vi "Read TDM Event Data.vi"() -> ()   [LabVIEW 2023]
doc: "Reads the data written by the Write TDM Event Data.vi example."
uses:
  <vilib>/Platform/storage/lvStorage.llb/_openFunction.ctl
  <vilib>/Platform/storage/lvStorage.llb/_openStorageWithRootAutoDetect.vi
  <vilib>/Platform/storage/lvStorage.llb/xStorage/xStorageSupp/ErrorOut.vi
  <vilib>/Platform/storage/lvStorage.llb/_queryPropPoly.vi
  <vilib>/Platform/storage/lvStorage.llb/_queryPropString.vi
  <vilib>/Platform/storage/lvStorage.llb/_queryGenericObjects.vi
  <vilib>/Platform/storage/lvStorage.llb/_loadAllDdt.vi
  <vilib>/Platform/storage/lvStorage.llb/_loadAllString.vi
  <vilib>/Platform/storage/Storage.llb/Get Object Info.vi
  <vilib>/Platform/storage/Storage.llb/__closeStorageFromObject.vi
  <vilib>/Platform/storage/lvStorage.llb/xStorage/Open Data Storage/Open Data Storage.xnode
  <vilib>/Platform/storage/lvStorage.llb/xStorage/Read Data/Read Data.xnode
  <vilib>/Platform/storage/lvStorage.llb/xStorage/Close Data Storage/Close Data Storage.xnode
panel:
  out "Events":string[][](table)
  out "Data":dynamicdata(graph)
  out "Histogram Results":dynamicdata(graph)
  # "Overview: Demonstrates the use of the DataPlugin Express VIs to read event data from a TDM file.\nRequirements: Windows\nInstructions:\n1. Make sure you have already run Write TDM Event Data.vi.\n2. Run this VI. The contents of the TDM file will be displayed below.\n3. Delete the TDM file (located at [LabVIEW Data]\\Example Event File.tdm) when you are done."
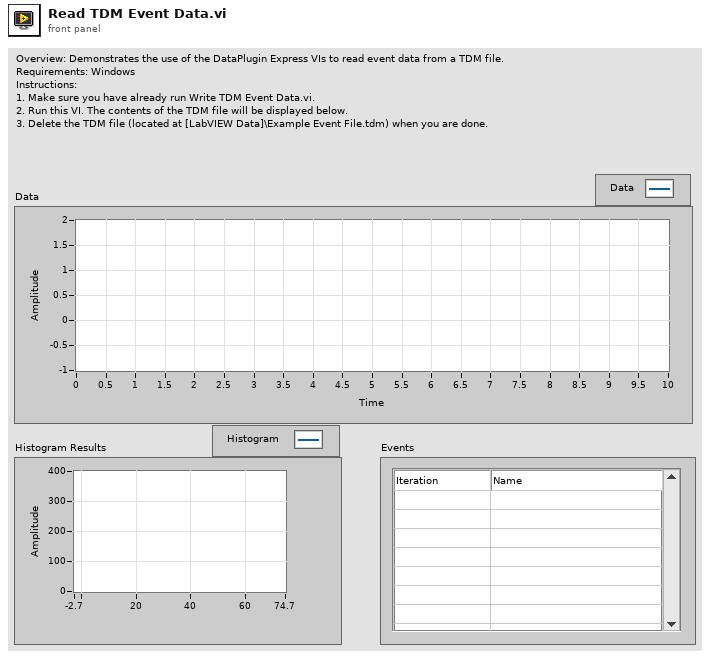
[diagram p1: front panel]
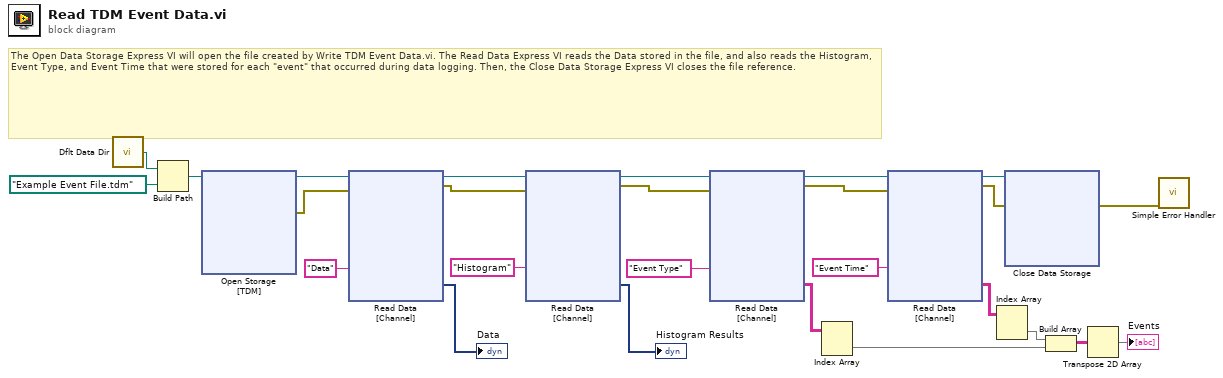
[diagram p0: block diagram]
diagram:
  # "The Open Data Storage Express VI will open the file created by Write TDM Event Data.vi. The Read Data Express VI reads the Data stored in the file, and also reads the Histogram, Event Type, and Event Time that were stored for each \"event\" that occurred during data logging. Then, the Close Data Storage Express VI closes the file reference."
  n1 = call <vilib>:"Dflt Data Dir.vi"() -> ("App:Default Data Directory"=w8:path)
  n2 = Build Path(base path=w8, name or relative path=path "Example Event File.tdm" ("default name")) -> (appended path=w7:path)
  n3 = xnode "Open Storage\n[TDM]"("file path"=w7) -> ("storage refnum (file)"=w13:refnum<k20>, "error out"=w12:errorcluster)  [unwired: 2 in, 3 out]
  n4 = xnode "Read Data\n[Channel]"("Name"="Data" ("registertxt3"), "storage refnum (file)"=w13, "error in"=w12) -> ("Signal"=→"Data":dynamicdata, "storage refnum (file) out"=w25:refnum<k20>, "error out"=w24:errorcluster)  [unwired: 1 out]
  n5 = xnode "Read Data\n[Channel]"("Name"="Histogram" ("name"), "storage refnum (file)"=w25, "error in"=w24) -> ("Signal"=→"Histogram Results":dynamicdata, "storage refnum (file) out"=w22:refnum<k20>, "error out"=w21:errorcluster)  [unwired: 1 out]
  n6 = xnode "Read Data\n[Channel]"("Name"="Event Type" ("name"), "storage refnum (file)"=w22, "error in"=w21) -> ("Signal"=w17:string[][], "storage refnum (file) out"=w19:refnum<k20>, "error out"=w18:errorcluster)  [unwired: 1 out]
  n7 = Index Array(array=w17) -> (element=w10:string[])  [unwired: 2 in]
  n8 = xnode "Read Data\n[Channel]"("Name"="Event Time" ("name"), "storage refnum (file)"=w19, "error in"=w18) -> ("Signal"=w16:string[][], "storage refnum (file) out"=w15:refnum<k20>, "error out"=w14:errorcluster)  [unwired: 1 out]
  n9 = Index Array(array=w16) -> (element=w2:string[])  [unwired: 2 in]
  n10 = xnode "Close Data Storage\n"("storage refnum (file)"=w15, "error in (no error)"=w14) -> ("error out"=w1:errorcluster)  [unwired: 1 out]
  n11 = Build Array(w2, w10) -> (w11:string[][])
  n12 = Transpose 2D Array(2D array=w11) -> (transposed array=→"Events":string[][])
  n13 = call <vilib>:"Simple Error Handler.vi"("error in (no error)"=w1) -> ()  [unwired: 4 in, 5 out]
